vi "Arduino Network Device Scan.vi"(2 "Resource index":i32) -> (0 "Network device table":string[][](table))   [LabVIEW 2016]
uses:
  Instrument drivers/Arduino/ctls_and_globals/Arduino tx msg cluster.ctl
  Instrument drivers/Arduino/ctls_and_globals/Arduino Global.vi
panel:
  in  "End addr.":u8=255
  in  "Start addr.":u8=1 min=1
  out "Current address":i32(slide) scale=0.0..255.0
  # "PN 12/06/2014"
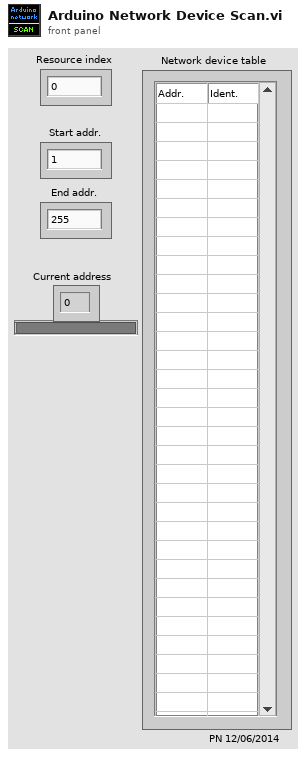
[diagram p1: front panel]
types:
  T1 = typedef "Arduino Config & resource typedef.ctl" = cluster{"VISA resource name":refnum<visa-resource-name>, "baud rate (bps)":u32, "timeout (ms)":u32, "data bits":u16, "parity":enum16{"None", "Odd", "Even", "Mark", "Space"}, "stop bits (10: 1 bit)":u16, "flow control":u16, "termination char (hex)":u8, "Enable Termination Char":bool, "byte count":u32, "Resource locked?":bool}
  T2 = typedef "Arduino tx msg cluster.ctl" = cluster{"dest":u8, "A/D/C/I":string, "R/W":string, "chan":u8, "val (float)":sgl}
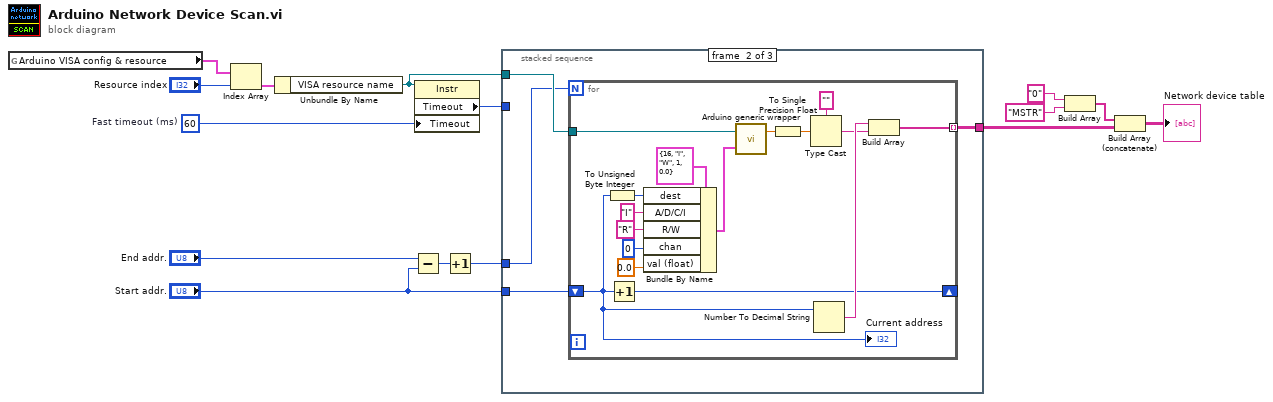
[diagram p0: block diagram]
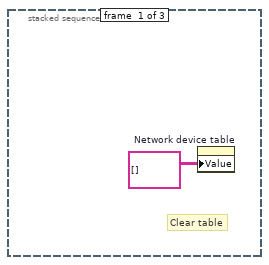
[diagram p2: hidden frame]
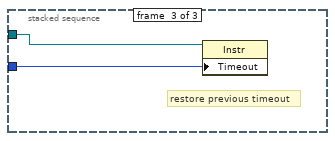
[diagram p3: hidden frame]
diagram:
  w15 = u32 60  # Fast timeout (ms)
  n1 = global read "Arduino Global.vi" "Arduino VISA config & resource"() -> (w11:T1[])
  n2 = Index Array(array=w11, index="Resource index") -> (element=w10:T1)
  n3 = Unbundle By Name(w10) -> ("VISA resource name"=w13:refnum<visa-resource-name>)
  n4 = Subtract(x="End addr.", y="Start addr.") -> (x-y=w2:u8)
  n5 = property class="Instr"(reference=w13, "Timeout"=w15) -> ("Timeout"=w14:u32)  [unwired: 1 in, 2 out]
  n6 = Increment(x=w2) -> (x+1=w1:u8)
  n7 = stacked-sequence {
    tunnel: w14 -> [_ _ w38]
    tunnel: w13 -> [_ w20 w37]
    tunnel: [_ w19 _] -> w6
    tunnel: "Start addr." -> [_ w18 _]
    tunnel: w1 -> [_ w17 _]
    frame #0 {
      # "Clear table"
      n8 = property on="Network device table" class="Tbl (strict)"("Value"=string[][] [] ("Network device table")) -> ()  [unwired: 2 in, 2 out]
    }
    frame #1 {
      n9 = for {
        N: w17 -> [_]
        tunnel: w20 -> [w26]
        tunnel: [w23] -> w19 mode=indexing
        shift-right: [w21] -> _
        shift-left: w18 -> [w22]
        n10 = To Unsigned Byte Integer(number=w22) -> (unsigned 8bit integer=w34:u8)
        n11 = Increment(x=w22) -> (x+1=w21:u8)
        n12 = Bundle By Name(cluster=T2 {"dest"=16, "A/D/C/I"="I", "R/W"="W", "chan"=1, "val (float)"=0.0} ("Tx msg cluster"), "dest"=w34, "A/D/C/I"="I" ("A/D/C"), "R/W"="R", "chan"=u8 0, "val (float)"=sgl 0.0) -> (w30:T2)
        n13 = call "Arduino generic wrapper.vi"("Tx msg cluster"=w30, "Port name"=w26) -> ("Output"=w28:dbl)  [unwired: 1 out]
        n14 = To Single Precision Float(number=w28) -> (single precision float=w27:sgl)
        n15 = Type Cast(type="", x=w27) -> (*(type *) &x=w24:string)
        n16 = Number To Decimal String(number=w22) -> (decimal integer string=w25:string)  [unwired: 1 in]
        n17 = Build Array(w25, w24) -> (w23:string[])
        "Current address" <- w22
      }
    }
    frame #2 {
      # "restore previous timeout"
      n18 = property class="Instr"(reference=w37, "Timeout"=w38) -> ()  [unwired: 1 in, 2 out]
    }
  }
  n19 = Build Array("0", "MSTR") -> (w7:string[])
  n20 = Build Array (concatenate)(w7, w6) -> (→"Network device table":string[][])
